vi "Trajectory_Equals.vi"(9 "other TRAJECTORY":T1 {"States"."POSE"."ROTATION"."SIN" format="%13.4f"; "States"."POSE"."ROTATION"."COS" format="%13.4f"; "States"."POSE"."ROTATION"."VALUE" format="%13.4f"; "States"."POSE"."TRANSLATION"."Y" format="%14.3f"; "States"."POSE"."TRANSLATION"."X" format="%14.3f"; "TotalTImeSecs" format="%20.3f"}, 11 "TRAJECTORY":T1 {"States"."POSE"."ROTATION"."SIN" format="%13.4f"; "States"."POSE"."ROTATION"."COS" format="%13.4f"; "States"."POSE"."ROTATION"."VALUE" format="%13.4f"; "States"."POSE"."TRANSLATION"."Y" format="%14.3f"; "States"."POSE"."TRANSLATION"."X" format="%14.3f"; "TotalTImeSecs" format="%20.3f"}) -> (3 "Equals":bool)   [LabVIEW 2019, in "Trajectory_Library.lvlib"]
doc: "Determines if two trajectories are equal.\n\nParameters:\n - Trajectory - Trajectory data structure\n - Other Trajectory - Trajectory data structure\n\nReturns:\n - Equals - boolean indicating if the two trajectories are equal."
uses:
  Trajectory_Library.lvlib
  TypeDef/TRANSLATION2D.ctl
  TypeDef/ROTATION2D.ctl
  TypeDef/POSE2D.ctl
  TypeDef/TRAJ_STATE.ctl
  TypeDef/TRAJECTORY.ctl
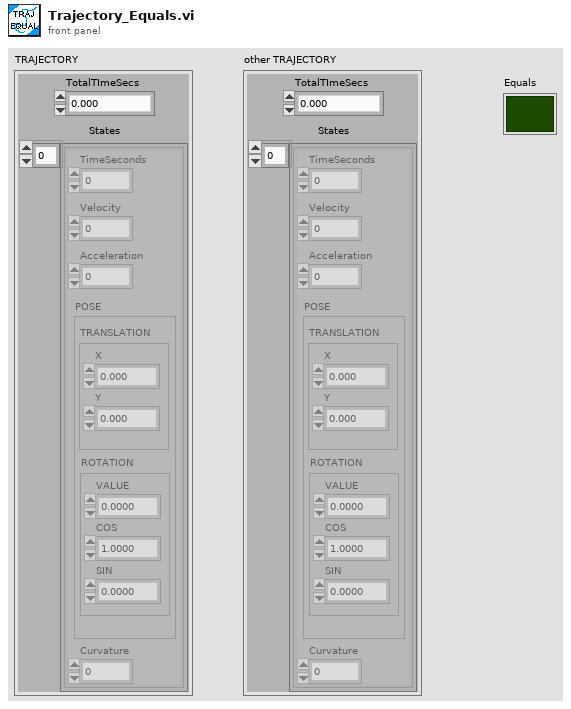
[diagram p1: front panel]
types:
  T1 = typedef "Trajectory_Library.lvlib/TRAJECTORY.ctl" = cluster{"TotalTImeSecs":dbl, "States":T2[]}
  T2 = typedef "Trajectory_Library.lvlib/TRAJ_STATE.ctl" = cluster{"TimeSeconds":dbl, "Velocity":dbl, "Acceleration":dbl, "POSE":T3, "Curvature":dbl}
  T3 = typedef "Trajectory_Library.lvlib/POSE2D.ctl" = cluster{"TRANSLATION":T4, "ROTATION":T5}
  T4 = typedef "Trajectory_Library.lvlib/TRANSLATION2D.ctl" = cluster{"X":dbl, "Y":dbl}
  T5 = typedef "Trajectory_Library.lvlib/ROTATION2D.ctl" = cluster{"VALUE":dbl, "COS":dbl, "SIN":dbl}
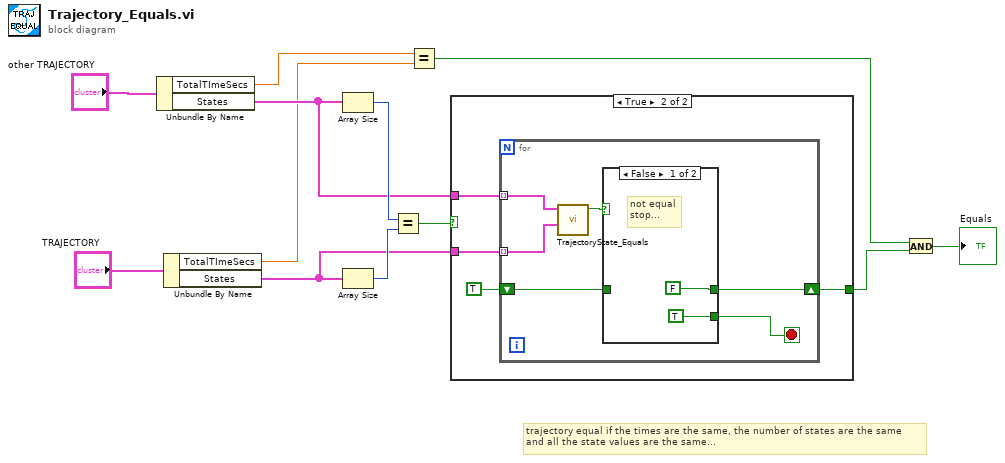
[diagram p0: block diagram]
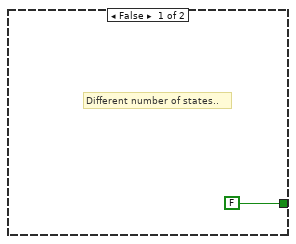
[diagram p2: hidden frame]
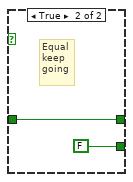
[diagram p3: hidden frame]
diagram:
  # "trajectory equal if the times are the same, the number of states are the same\nand all the state values are the same..."
  n1 = Unbundle By Name("other TRAJECTORY") -> ("TotalTImeSecs"=w4:dbl, "States"=w6:T2[])
  n2 = Unbundle By Name("TRAJECTORY") -> ("TotalTImeSecs"=w5:dbl, "States"=w7:T2[])
  n3 = Array Size(array=w6) -> (size(s)=w10:i32)
  n4 = Array Size(array=w7) -> (size(s)=w9:i32)
  n5 = Equal?(x=w10, y=w9) -> (x = y?=w8:bool)
  n6 = Equal?(x=w4, y=w5) -> (x = y?=w2:bool)
  n7 = case shown="True" w8 {
    tunnel: [FALSE w16] -> w3
    tunnel: w7 -> [_ w15]
    tunnel: w6 -> [_ w14]
    frame False {
      # "Different number of states.."
    }
    frame True {
      n8 = for {
        shift-right: [w19] -> w16
        shift-left: TRUE -> [w20]
        tunnel: w15 -> [w22] mode=indexing
        tunnel: w14 -> [w23] mode=indexing
        stop <- w18 stop-if-true
        n9 = call "TrajectoryState_Equals.vi"("Other TRAJ_STATE"=w22, "TRAJ_STATE"=w23) -> ("Equals"=w21:bool)  [unwired: 9 in]
        n10 = case shown="False" w21 {
          tunnel: w20 -> [_ w27]
          tunnel: [FALSE w27] -> w19
          tunnel: [TRUE FALSE] -> w18
          frame False {
            # "not equal\nstop..."
          }
          frame True {
            # "Equal\nkeep\ngoing"
          }
        }
      }
    }
  }
  n11 = And(x=w2, y=w3) -> (x .and. y?=→"Equals":bool)
